vi "Set SDO Response.vi"(10 "SDO Response":refnum<notifier>, 11 "CANopen in":refnum<class "CANopen.lvclass">) -> (3 "CANopen out":refnum<class "CANopen.lvclass">)   [LabVIEW 2024, in "canopen.lvlib" / "CANopen.lvclass"]
uses:
  CANopen.lvclass
  CANopen.lvclass/CANopen.ctl
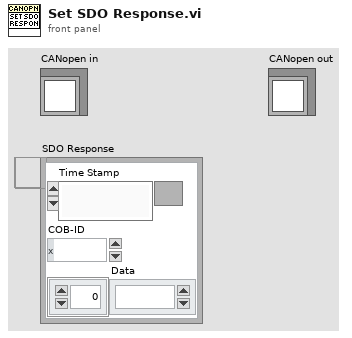
[diagram p1: front panel]
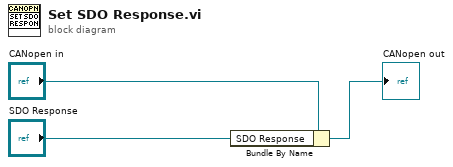
[diagram p0: block diagram]
diagram:
  n1 = Bundle By Name(cluster="CANopen in", "SDO Response"="SDO Response") -> (→"CANopen out":refnum<class "CANopen.lvclass">)
